vi "StringToI32(cast).vi"(1 "String":string) -> (0 "I32":i32)   [LabVIEW 2012]
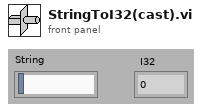
[diagram p1: front panel]
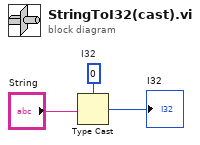
[diagram p0: block diagram]
diagram:
  w2 = 0  # I32
  n1 = Type Cast(type=w2, x="String") -> (*(type *) &x=→"I32":i32)
